vi "GetParametrAddress.vi"(8 "error in (no error)":errorcluster, 10 "Адрес параметра":u16 format="%04x", 11 "StepMotor in":refnum<class "StepMotor.lvclass">) -> (0 "error out":errorcluster, 2 "Значение":dbl, 3 "StepMotor out":refnum<class "StepMotor.lvclass">)   [LabVIEW 2010, in "StepMotor.lvclass"]
uses:
  StepMotor.lvclass
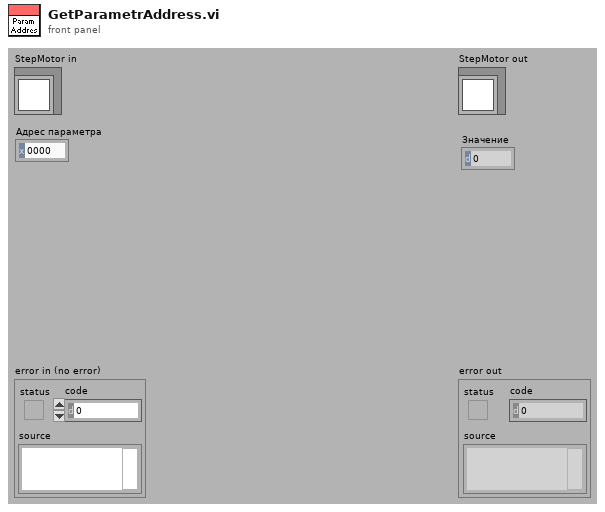
[diagram p1: front panel]
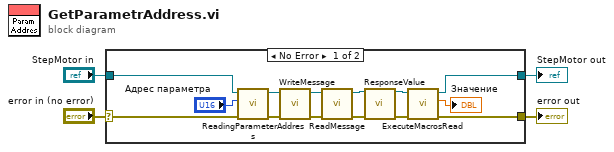
[diagram p0: block diagram]
diagram:
  n1 = case shown="No Error" "error in (no error)" {
    selector: "error in (no error)" -> [w15 w20]
    tunnel: [w10 w20] -> w3
    tunnel: [w11 w19] -> w1
    tunnel: "StepMotor in" -> [w17 w19]
    frame No Error {
      n2 = call "ReadingParameterAddress.vi"("error in (no error)"=w15, "Адрес параметра"="Адрес параметра", "StepMotor in"=w17) -> ("error out"=w7:errorcluster, "StepMotor out"=w8:refnum<class "StepMotor.lvclass">)  [unwired: 7 in]
      n3 = call-dynamic "WriteMessage.vi"("error in (no error)"=w7, "StepMotor in"=w8) -> ("error out"=w18:errorcluster, "StepMotor out"=w16:refnum<class "StepMotor.lvclass">)  [unwired: 8 in]
      n4 = call-dynamic "ReadMessage.vi"("error in (no error)"=w18, "StepMotor in"=w16) -> ("error out"=w5:errorcluster, "StepMotor out"=w6:refnum<class "StepMotor.lvclass">)  [unwired: 8 in]
      n5 = call-dynamic "ResponseValue.vi"("StepMotor in"=w6, "error in (no error)"=w5) -> ("StepMotor out"=w13:refnum<class "StepMotor.lvclass">, "error out"=w12:errorcluster)  [unwired: 12 in]
      n6 = call "ExecuteMacrosRead.vi"("error in (no error)"=w12, "StepMotor in"=w13) -> ("error out"=w10:errorcluster, "Значение"=→"Значение":dbl, "StepMotor out"=w11:refnum<class "StepMotor.lvclass">)  [unwired: 7 in]
    }
    frame Error {
    }
  }
  "error out" <- w3
  "StepMotor out" <- w1
